vi "SOLOCITAR MERCANCIA.vi"(8 "error in (no error)":errorcluster, 10 "appended array":string[][](array[string]), 11 "CAFE_MEX_ESP in":refnum<class "CAFE_MEX_ESP.lvclass">) -> (0 "error out":errorcluster, 3 "CAFE_MEX_ESP out":refnum<class "CAFE_MEX_ESP.lvclass">)   [LabVIEW 2019, in "CAFE_MEX_ESP.lvlib" / "CAFE_MEX_ESP.lvclass"]
uses:
  CAFE_MEX_ESP.lvclass
  CAFE_MEX_ESP.lvclass/CAFE_MEX_ESP.ctl
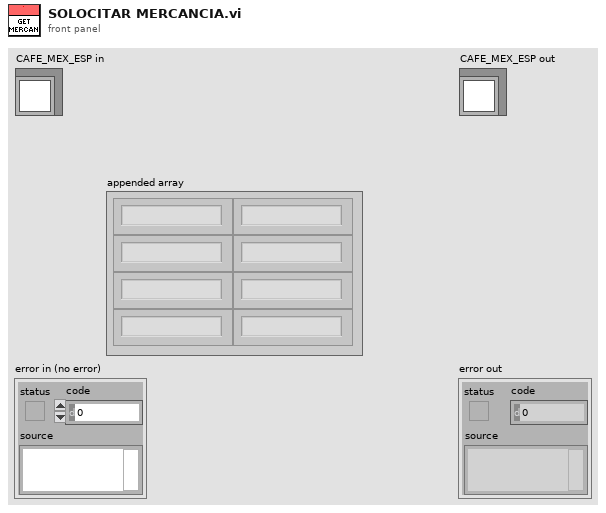
[diagram p1: front panel]
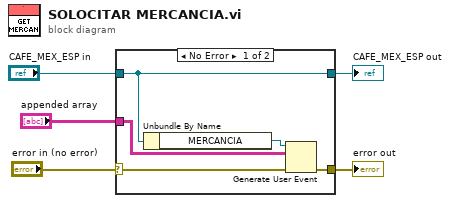
[diagram p0: block diagram]
diagram:
  n1 = case shown="No Error" "error in (no error)" {
    selector: "error in (no error)" -> [w7 w12]
    tunnel: [w6 w12] -> w4
    tunnel: [w10 w11] -> w2
    tunnel: "CAFE_MEX_ESP in" -> [w10 w11]
    tunnel: "appended array" -> [w8 _]
    frame No Error {
      n2 = Unbundle By Name(w10) -> ("MERCANCIA"=w9:refnum<user-event>)
      n3 = Generate User Event(user event=w9, event data cluster=w8, error in=w7) -> (error out=w6:errorcluster)  [unwired: 1 in, 1 out]
    }
    frame Error {
    }
  }
  "error out" <- w4
  "CAFE_MEX_ESP out" <- w2
